vi "Basic_test.vi"(4 "Frecuencia":u32(slide) scale=0.0..60.0) -> ()   [LabVIEW 2011]
uses:
  mbed/Transport Mechanisms/HTTPRPC/HTTPRPC.lvclass
  mbed/mbed Interface/RPCFunction/RPCFunction.lvclass
panel:
  out "output":string
  in  "Vout":dbl(slide) scale=-10.0..10.0
  in  "stop":bool
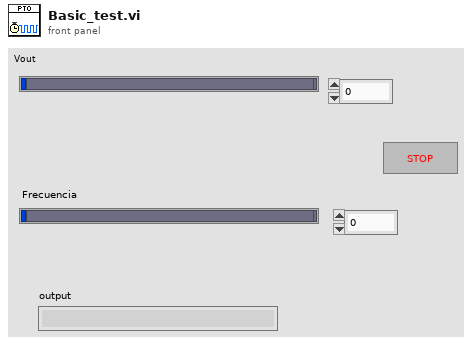
[diagram p1: front panel]
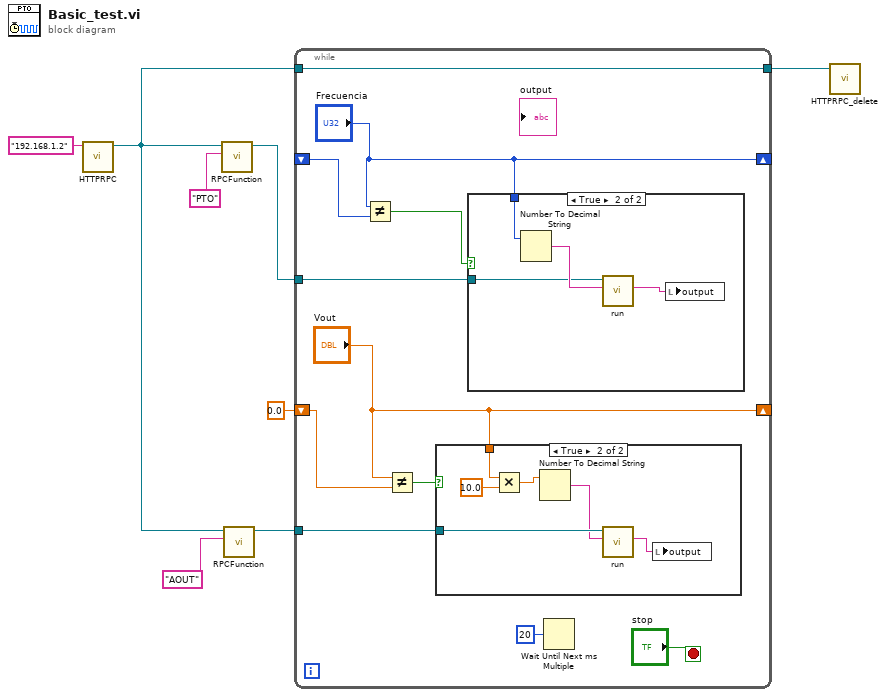
[diagram p0: block diagram]
diagram:
  n1 = call "HTTPRPC.vi"("Address"="192.168.1.2") -> ("mbed.lvclass"=w1:refnum<class "mbed.lvclass">)  [unwired: 7 in, 1 out]
  n2 = call "RPCFunction.vi"("Existing Obj Name"="PTO", "mbed_LVLibrary.lvlib:mbed.lvclass"=w1) -> ("mbed_LVLibrary.lvlib:Packet.lvclass 2"=w3:refnum<class "RPCFunction.lvclass">)  [unwired: 7 in, 2 out]
  n3 = call "RPCFunction.vi"("Existing Obj Name"="AOUT", "mbed_LVLibrary.lvlib:mbed.lvclass"=w1) -> ("mbed_LVLibrary.lvlib:Packet.lvclass 2"=w2:refnum<class "RPCFunction.lvclass">)  [unwired: 7 in, 2 out]
  n4 = while {
    tunnel: [w17] -> w5
    tunnel: w1 -> [w17]
    shift-right: ["Vout"] -> _
    shift-left: 0.0 ("PTO") -> [w16]
    shift-right: ["Frecuencia"] -> _
    shift-left: _ -> [w14]
    tunnel: w3 -> [w11]
    tunnel: w2 -> [w9]
    stop <- "stop" stop-if-true
    n5 = Not Equal?(x="Frecuencia", y=w14) -> (x != y?=w13:bool)
    n6 = Not Equal?(x="Vout", y=w16) -> (x != y?=w15:bool)
    n7 = case shown="True" w15 {
      tunnel: w9 -> [_ w29]
      tunnel: "Vout" -> [_ w27]
      frame False {
      }
      frame True {
        n8 = Multiply(x=w27, y=10.0) -> (x*y=w25:dbl)
        n9 = Number To Decimal String(number=w25) -> (decimal integer string=w24:string)  [unwired: 1 in]
        n10 = call "run.vi"("Input"=w24, "Packet in"=w29) -> ("Output"=w28:string)  [unwired: 7 in, 2 out]
        n11 = local write "output"(w28) -> ()
      }
    }
    n12 = case shown="True" w13 {
      tunnel: "Frecuencia" -> [_ w23]
      tunnel: w11 -> [_ w21]
      frame False {
      }
      frame True {
        n13 = Number To Decimal String(number=w23) -> (decimal integer string=w22:string)  [unwired: 1 in]
        n14 = call "run.vi"("Input"=w22, "Packet in"=w21) -> ("Output"=w20:string)  [unwired: 7 in, 2 out]
        n15 = local write "output"(w20) -> ()
      }
    }
    n16 = Wait Until Next ms Multiple(millisecond multiple=u32 20) -> ()  [unwired: 1 out]
  }
  n17 = call "HTTPRPC_delete.vi"("mbed_LVLibrary.lvlib:mbed.lvclass"=w5) -> ()  [unwired: 9 in, 1 out]
